vi "generalUI.vi"(11 "GeneralDisplay in":refnum<class "GeneralDisplay.lvclass">) -> ()   [LabVIEW 2017, in "GeneralDisplay.lvclass"]
uses:
  GeneralDisplay.lvclass
panel:
  out "GeneralDisplay out":refnum<class "GeneralDisplay.lvclass">
  out "Humidity":dbl(slide) scale=0.0..10.0
  out "Pressure":dbl(knob) scale=0.0..10.0
  out "Temperature":dbl(slide) scale=0.0..10.0
  out "error out":errorcluster
  in  "error in (no error)":errorcluster
  # "General Display"
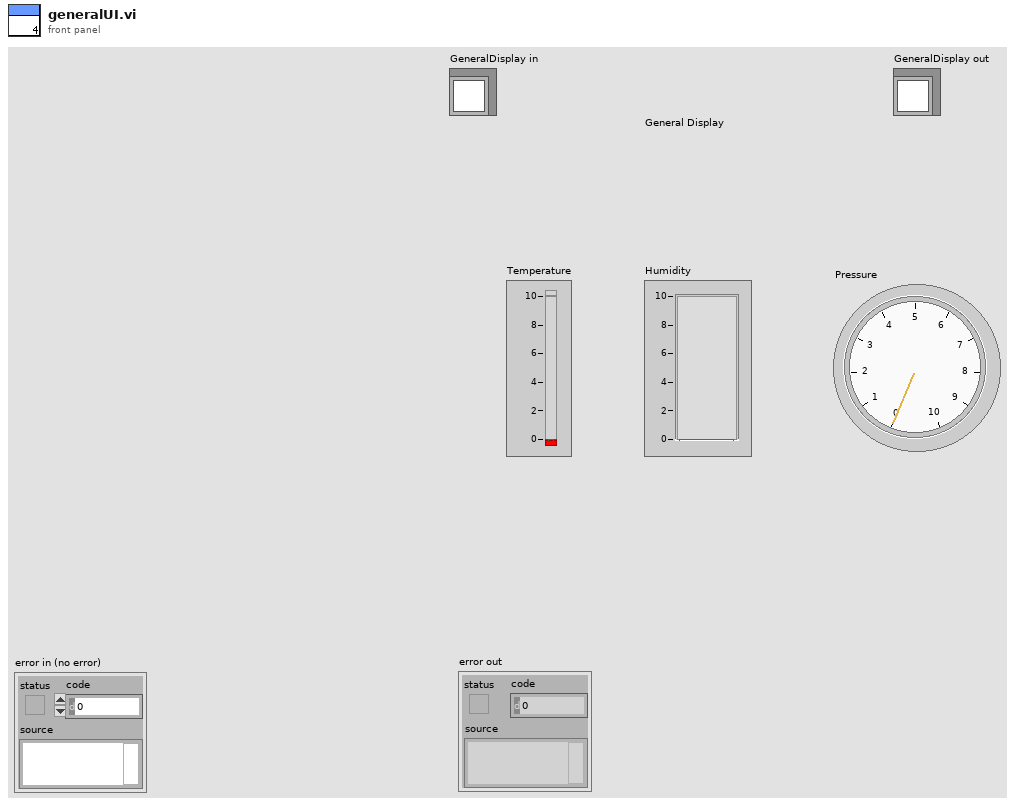
[diagram p1: front panel]
types:
  T1 = enum16{"Always On", "Always Off", "Off While Running"}
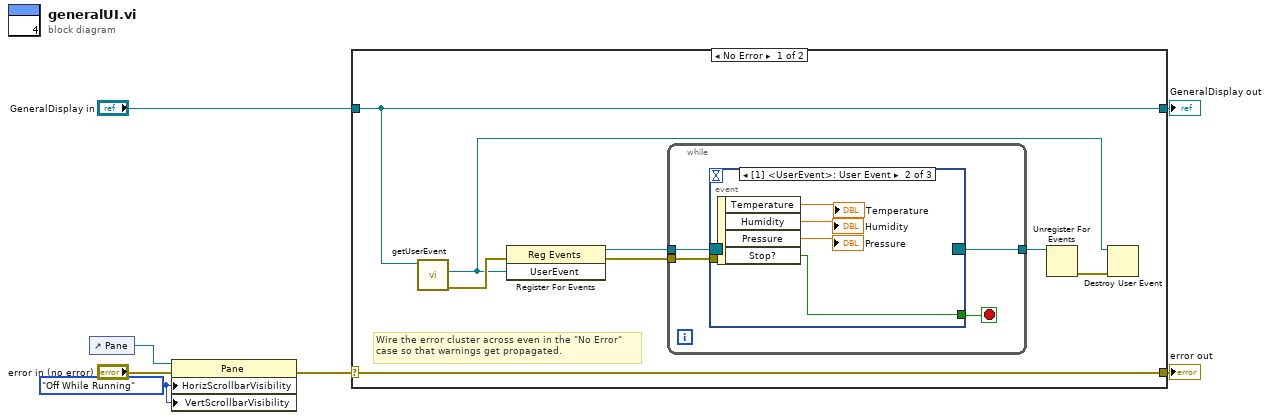
[diagram p0: block diagram]
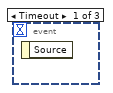
[diagram p2: hidden frame]
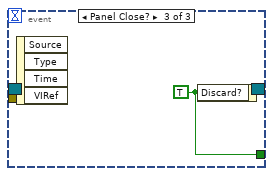
[diagram p3: hidden frame]
diagram:
  w2 = T1."Off While Running" ("Horizontal Scrollbar Visibility")
  n1 = control-ref of="Pane"() -> (w1:refnum<vi>)
  n2 = property class="Pane"(reference=w1, error in="error in (no error)", "HorizScrollbarVisibility"=w2, "VertScrollbarVisibility"=w2) -> (error out=w3:errorcluster)  [unwired: 1 out]
  n3 = case shown="No Error" w3 {
    selector: w3 -> [w15 w26]
    tunnel: [w15 w26] -> w6
    tunnel: [w11 w25] -> w4
    tunnel: "GeneralDisplay in" -> [w11 w25]
    frame No Error {
      # "Wire the error cluster across even in the \"No Error\"\ncase so that warnings get propagated."
      n4 = call-dynamic "getUserEvent.vi"("GeneralDisplay in"=w11) -> ("error out"=w13:errorcluster, "UserEvent"=w8:refnum<user-event>)  [unwired: 8 in, 1 out]
      n5 = register-events(error in=w13, w8) -> (reference out=w14:refnum<event-registration>, error out=w12:errorcluster)  [unwired: 1 in]
      n6 = while {
        tunnel: w14 -> [w19]
        tunnel: w12 -> [w18]
        tunnel: [w16] -> w10
        stop <- w17 stop-if-true
        n7 = event shown="[1] <UserEvent>: User Event" {
          selector: w19 -> [_ _ _]
          dyn-events: [_ _ _] -> w16
          timeout: _ -> [_ _ _]
          tunnel: w18 -> [_ _ _]
          tunnel: [_ w20 w24] -> w17
          event Timeout {
            n8 = event-data() -> ()  [unwired: 1 in, 1 out]
          }
          event User Event {
            n9 = event-data() -> ("Temperature"=→"Temperature":dbl, "Humidity"=→"Humidity":dbl, "Pressure"=→"Pressure":dbl, "Stop?"=w20:bool)  [unwired: 1 in]
          }
          event Panel Close? {
            w24 = TRUE ("Discard?")
            n10 = event-data() -> ()  [unwired: 1 in, 4 out]
            n11 = event-data("Discard?"=w24) -> ()  [unwired: 1 in, 1 out]
          }
        }
      }
      n12 = Unregister For Events(event registration refnum=w10) -> (error out=w9:errorcluster)  [unwired: 1 in]
      n13 = Destroy User Event(user event=w8, error in=w9) -> ()  [unwired: 1 out]
    }
    frame Error {
    }
  }
  "error out" <- w6
  "GeneralDisplay out" <- w4
